vi "Add Default Free.vi"(8 "error in (no error)":errorcluster, 10 "ToModBus":bool, 11 "Volt In":refnum<class "Voltage.lvclass">) -> (0 "error out":errorcluster, 3 "Volt Out":refnum<class "Voltage.lvclass">)   [LabVIEW 2012, in "Measurement Channels.lvlib" / "Voltage.lvclass"]
uses:
  Voltage.lvclass
  Class Channel/Channel.lvclass
  Class Channel/Write Unit_EU.vi
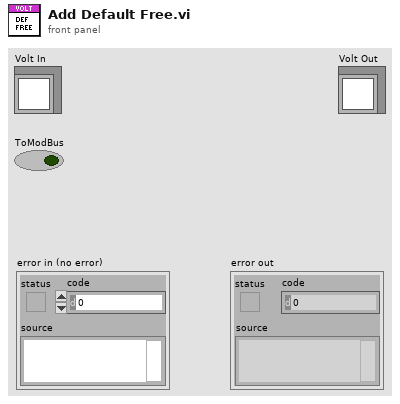
[diagram p1: front panel]
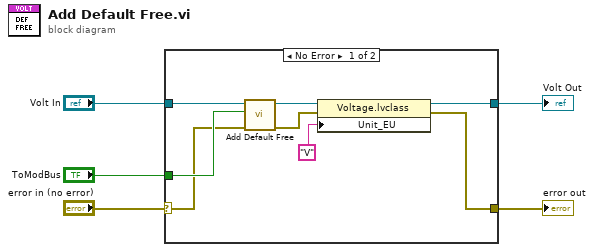
[diagram p0: block diagram]
diagram:
  n1 = case shown="No Error" "error in (no error)" {
    selector: "error in (no error)" -> [w11 w15]
    tunnel: [w9 w14] -> w5
    tunnel: [w6 w15] -> w4
    tunnel: "Volt In" -> [w13 w14]
    tunnel: "ToModBus" -> [w12 _]
    frame No Error {
      n2 = call-parent "Add Default Free.vi"("error in (no error)"=w11, "ToModBus"=w12, "Channel in"=w13) -> ("error out"=w8:errorcluster, "Channel out"=w10:refnum<class "Voltage.lvclass">)  [unwired: 7 in]
      n3 = property class="Voltage.lvclass"(reference=w10, error in=w8, "Unit_EU"="V") -> (reference out=w9:refnum<class "Voltage.lvclass">, error out=w6:errorcluster)
    }
    frame Error {
    }
  }
  "Volt Out" <- w5
  "error out" <- w4
